vi "PicoStatus2.vi"(5 "PICO source":string, 6 "Error in":errorcluster, 7 "PICO_STATUS in":T1, 8 "PICO STATUS":u32) -> (0 "error out":errorcluster, 1 "PICO_STATUS out":T1)   [LabVIEW 2017]
doc: "This VI checks the PICO_STATUS value returned by calls to the PICO API. If it returns an error, the status member of the \"PICO_STATUS in\" cluster is set to 'true' and the error code and source are set.\nIt also sets the error cluster to BFFC0F80 - ERROR: PICO STATUS API Error (used for instrument drivers) if PICO_STATUS value is not an error value.\nThese default values can be change in the vi."
panel:
  in  "code":i32=-1074000000 format="%x"
  in  "source":string="ERROR: PICO STATUS API Error"
  # "ERROR: Instrument Defined Error"
  # "Set default value for a PICO error"
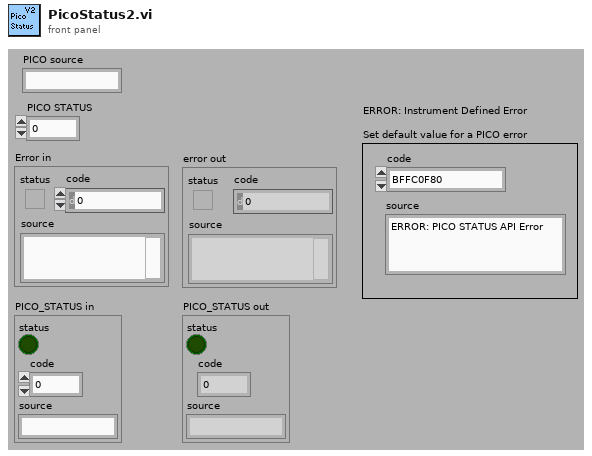
[diagram p1: front panel]
types:
  T1 = cluster{"status":bool, "code":u32, "source":string}
  T2 = cluster{"status":bool, "code":u32, "source":string}[]
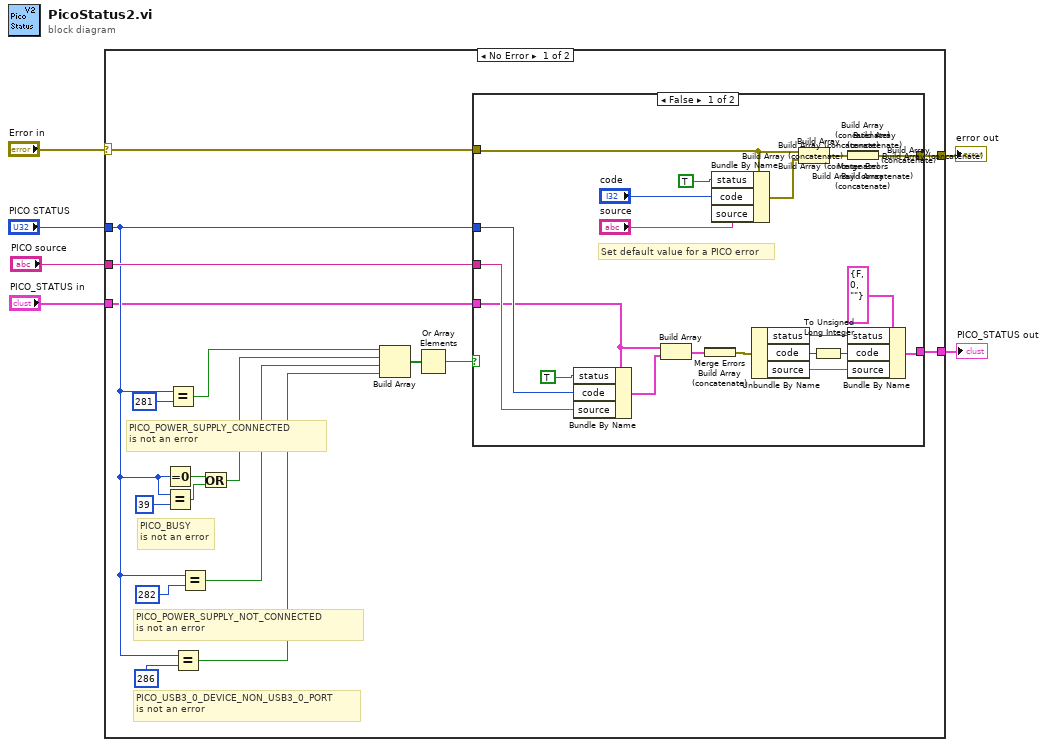
[diagram p0: block diagram]
diagram:
  n1 = case shown="No Error" "Error in" {
    selector: "Error in" -> [w7 w58]
    tunnel: [w24 w58] -> w4
    tunnel: "PICO STATUS" -> [w11 _]
    tunnel: "PICO source" -> [w23 _]
    tunnel: [w9 w57] -> w3
    tunnel: "PICO_STATUS in" -> [w8 w57]
    frame No Error {
      # "PICO_USB3_0_DEVICE_NON_USB3_0_PORT\nis not an error"
      # "PICO_POWER_SUPPLY_CONNECTED \nis not an error"
      # "PICO_POWER_SUPPLY_NOT_CONNECTED \nis not an error"
      # "PICO_BUSY \nis not an error"
      n2 = Equal To 0?(x=w11) -> (x = 0?=w22:bool)
      n3 = Equal?(x=w11, y=u32 39) -> (x = y?=w21:bool)
      n4 = Equal?(x=w11, y=u32 281) -> (x = y?=w17:bool)
      n5 = Equal?(x=w11, y=u32 286) -> (x = y?=w10:bool)
      n6 = Equal?(x=w11, y=u32 282) -> (x = y?=w15:bool)
      n7 = Or(x=w22, y=w21) -> (x .or. y?=w16:bool)
      n8 = Build Array(w17, w16, w15, w10) -> (w14:bool[])
      n9 = Or Array Elements(Boolean array=w14) -> (logical OR=w13:bool)
      n10 = case shown="False" w13 {
        tunnel: w7 -> [w43 w56]
        tunnel: [w54 w56] -> w24
        tunnel: w11 -> [w39 _]
        tunnel: w23 -> [w38 _]
        tunnel: [w27 w55] -> w9
        tunnel: w8 -> [w37 w55]
        frame False {
          # "Set default value for a PICO error"
          n11 = Bundle By Name(cluster=w37, "status"=TRUE, "code"=w39, "source"=w38) -> (w40:T1)
          n12 = Build Array(w37, w40) -> (w28:T2)
          n13 = Build Array (concatenate)(w28) -> (w26:T2)
          n14 = Merge Errors(w26) -> (w30:errorcluster)
          n15 = Bundle By Name(cluster=w43, "status"=TRUE, "code"="code", "source"="source") -> (w42:errorcluster)
          n16 = Unbundle By Name(w30) -> ("status"=w31:bool, "code"=w34:i32, "source"=w32:string)
          n17 = Build Array(w43, w42) -> (w52:errorcluster[])
          n18 = To Unsigned Long Integer(number=w34) -> (unsigned 32bit integer=w33:u32)
          n19 = Build Array (concatenate)(w52) -> (w51:errorcluster[])
          n20 = Build Array (concatenate)(w51) -> (w50:errorcluster[])
          n21 = Build Array (concatenate)(w50) -> (w49:errorcluster[])
          n22 = Build Array (concatenate)(w49) -> (w48:errorcluster[])
          n23 = Build Array (concatenate)(w48) -> (w47:errorcluster[])
          n24 = Build Array (concatenate)(w47) -> (w46:errorcluster[])
          n25 = Build Array (concatenate)(w46) -> (w45:errorcluster[])
          n26 = Build Array (concatenate)(w45) -> (w44:errorcluster[])
          n27 = Build Array (concatenate)(w44) -> (w25:errorcluster[])
          n28 = Merge Errors(w25) -> (w54:errorcluster)
          n29 = Bundle By Name(cluster=T1 {"status"=FALSE, "code"=0, "source"=""} ("PICO_STATUS in"), "status"=w31, "code"=w33, "source"=w32) -> (w27:T1)
        }
        frame True {
        }
      }
    }
    frame Error {
    }
  }
  "error out" <- w4
  "PICO_STATUS out" <- w3
